vi "TriangleContinuityTest.vi"(6 "Pulse Positions Array":T1[](array[typedef]), 9 "Acq Block Number":i32, 10 "Waveforms":waveform(sgl)[](array[waveform]), 11 "Qbus in":refnum<class "Qbus.lvclass">) -> ()   [LabVIEW 2017]
uses:
  <vilib>/addons/Qbus/Qbus.lvclass
  <vilib>/addons/InsightCM/Utilities/Analysis/Shared/controls/PulsePositions.ctl
  <vilib>/addons/InsightCM/Utilities/Analysis/Shared/AnalysisHelper.lvlib
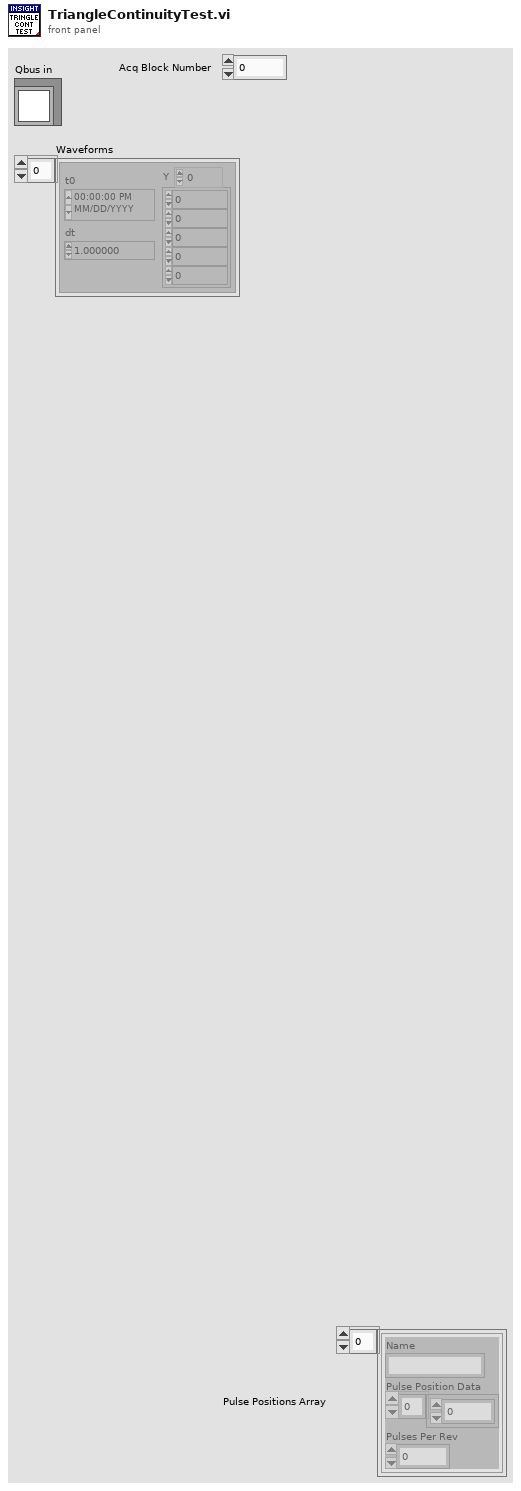
[diagram p1: front panel]
types:
  T1 = typedef "AnalysisHelper.lvlib/PulsePositions.ctl" = cluster{"Name":string, "Pulse Position Data":dbl[], "Pulses Per Rev":i32}
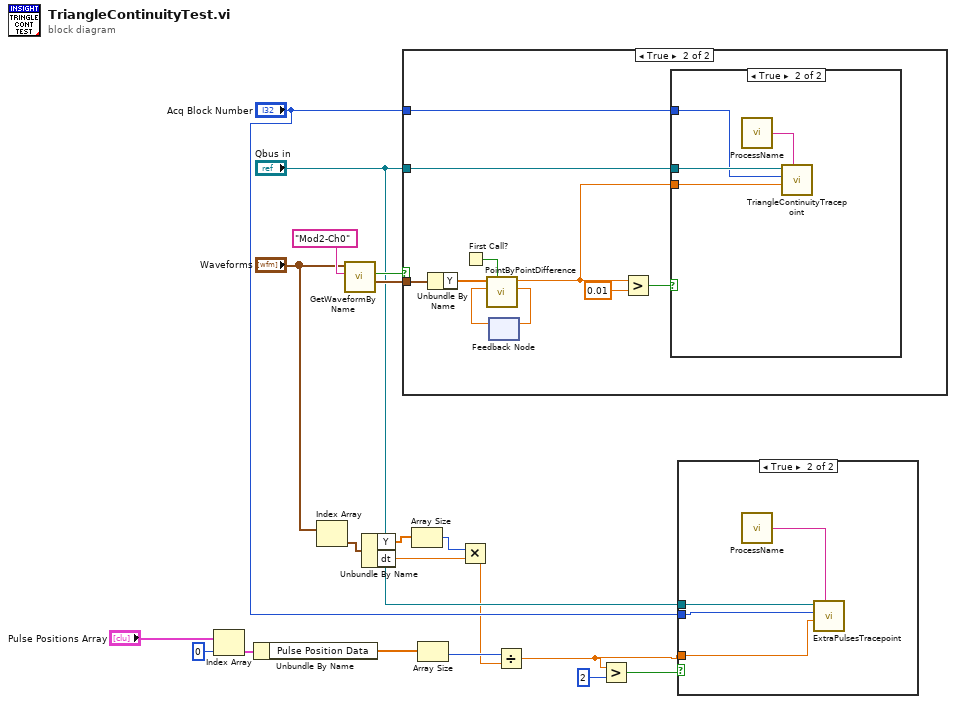
[diagram p0: block diagram]
diagram:
  n1 = Index Array(array="Pulse Positions Array", index=0) -> (element=w12:T1)
  n2 = Unbundle By Name(w12) -> ("Pulse Position Data"=w9:dbl[])
  n3 = Index Array(array="Waveforms") -> (element=w7:waveform(sgl))  [unwired: 1 in]
  n4 = call <vilib>:"GetWaveformByName.vi"("Channel Name"="Mod2-Ch0", "Acq Waveforms"="Waveforms") -> ("Waveform"=w18:waveform(sgl), "Found?"=w17:bool)  [unwired: 6 in, 2 out]
  n5 = Unbundle By Name(w7) -> ("Y"=w6:sgl[], "dt"=w4:dbl)
  n6 = case shown="True" w17 {
    tunnel: "Qbus in" -> [_ w29]
    tunnel: w18 -> [_ w27]
    tunnel: "Acq Block Number" -> [_ w22]
    frame False {
    }
    frame True {
      n7 = Unbundle By Name(w27) -> ("Y"=w28:sgl[])
      n8 = First Call?() -> (First Call?: T/F=w21:bool)
      n9 = feedback #1() -> (w25:dbl)  [unwired: 1 in]
      n10 = call <vilib>:"PointByPointDifference.vi"("reset?"=w21, "initial condition"=w25, "array"=w28) -> ("last point"=w26:dbl, "max difference"=w20:dbl)  [unwired: 6 in, 1 out]
      n11 = feedback-in #1(w26) -> ()
      n12 = Greater?(x=w20, y=0.01) -> (0:w23:bool)
      n13 = case shown="True" w23 {
        tunnel: w29 -> [_ w33]
        tunnel: w22 -> [_ w32]
        tunnel: w20 -> [_ w31]
        frame False {
        }
        frame True {
          n14 = call <vilib>:"ProcessName.vi"() -> ("ProcessName"=w30:string)  [unwired: 5 in]
          n15 = call <vilib>:"TriangleContinuityTracepoint.vi"("service name"=w30, "max difference"=w31, "Acq Block Number"=w32, "Qbus in"=w33) -> ()  [unwired: 7 in, 1 out]
        }
      }
    }
  }
  n16 = Array Size(array=w6) -> (size(s)=w5:i32)
  n17 = Array Size(array=w9) -> (size(s)=w3:i32)
  n18 = Multiply(x=w5, y=w4) -> (x*y=w2:dbl)
  n19 = Divide(x=w3, y=w2) -> (x/y=w1:dbl)
  n20 = Greater?(x=w1, y=2) -> (0:w10:bool)
  n21 = case shown="True" w10 {
    tunnel: "Qbus in" -> [_ w36]
    tunnel: "Acq Block Number" -> [_ w35]
    tunnel: w1 -> [_ w34]
    frame False {
    }
    frame True {
      n22 = call <vilib>:"ProcessName.vi"() -> ("ProcessName"=w37:string)  [unwired: 5 in]
      n23 = call <vilib>:"ExtraPulsesTracepoint.vi"("service name"=w37, "pulses"=w34, "Acq Block Number"=w35, "Qbus in"=w36) -> ()  [unwired: 7 in, 1 out]
    }
  }
